vi "Write First Call.vi"(8 "error in":errorcluster, 10 "First Call?":bool, 11 "STEP in":refnum<class "STEP.lvclass">) -> (0 "error out":errorcluster, 3 "STEP out":refnum<class "STEP.lvclass">)   [LabVIEW 2018, in "Sequence Composition.lvlib" / "STEP.lvclass"]
uses:
  STEP.lvclass
  STEP.lvclass/STEP.ctl
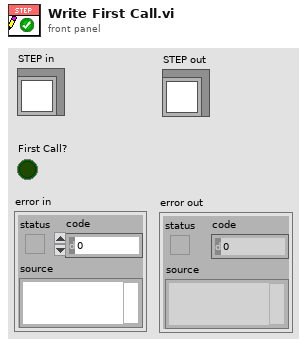
[diagram p1: front panel]
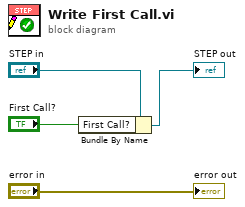
[diagram p0: block diagram]
diagram:
  n1 = Bundle By Name(cluster="STEP in", "First Call?"="First Call?") -> (→"STEP out":refnum<class "STEP.lvclass">)
  "error out" <- "error in"
